vi "_Yt06_Lock.vi"(11 "YTESTER测试数据":T1) -> (3 "YTESTER结论":T2)   [LabVIEW 2017]
doc: "VIClassID=YT_SSTEPFLAG_LOCK\nVIDescription=锁"
uses:
  YtCommon.lvlibp/yt`Step StepBaseInput.ctl
  YtCommon.lvlibp/yt`Step StepResult.ctl
  YtCommon.lvlibp/yt`Step TestData.ctl
  YtCommon.lvlibp/yt`Step System Queue.ctl
  Step`s VIs/YYLLGeneric/variable_W.ctl
  YtCommon.lvlibp/yt`Data-Ytester Type Data.ctl
  0f7d8788-236d-43a4-88cb-40465cf95507.vi
  b398933d-6113-41d7-8023-f37935ba96c7.vi
  <vilib>/Utility/error.llb/Clear Errors.vi
  YtCommon.lvlibp/yt`varSystemlib IO Read Variable.vi
  YtCommon.lvlibp
panel:
  in  "YTESTER开放参数":T4={"YTESTER_BaseInput"={"isTest"=TRUE, "isSkip"=FALSE, "StepName"="锁", "OnPass"=enum."Next", "OnFail"=enum."Terminate", "ReTestNumber"=0.0}, "解锁？"=FALSE, "锁名称"="Lock", "超时s"=-1.0}
  # "#yyll 首先这个必须是重入VI"
  # "YT_SSTEPFLAG_LOCK"
  # "#yyll 注意终止测试对解锁的影响"
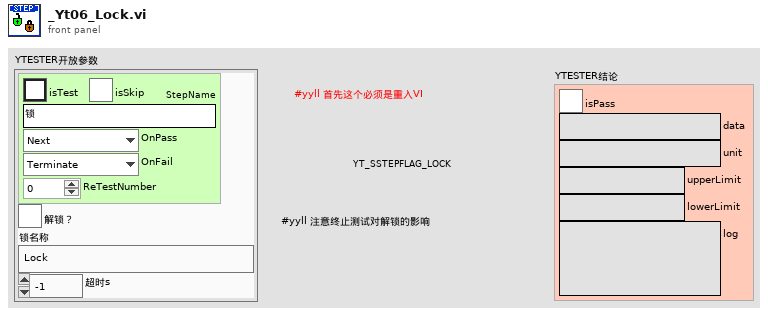
[diagram p1: front panel]
types:
  T1 = typedef "YtCommon.lvlibp/yt`Step TestData.ctl" = cluster{"Socket(From1)":i32, "SN":refnum<notifier>, "StopFlagRef":refnum<notifier>, "YT System Queue":refnum<queue>}
  T2 = typedef "YtCommon.lvlibp/yt`Step StepResult.ctl" = cluster{"isPass":bool, "data":string, "unit":string, "upperLimit":string, "lowerLimit":string, "log":string}
  T3 = typedef "YtCommon.lvlibp/yt`Step StepBaseInput.ctl" = cluster{"isTest":bool, "isSkip":bool, "StepName":string, "OnPass":enum16{"Next", "ToOVER", "Terminate"}, "OnFail":enum16{"Next", "ToOVER", "Terminate"}, "ReTestNumber":dbl}
  T4 = cluster{"YTESTER_BaseInput":T3, "解锁？":bool, "锁名称":string, "超时s":dbl}
  T5 = typedef "variable_W.ctl" = cluster{"YT_TYPE":T6, "TypeData":string[], "Tips":string}
  T6 = typedef "YtCommon.lvlibp/yt`Data-Ytester Type Data.ctl" = enum16{"NULL", "NUM", "BOOL", "TXT", "ENUM", "TIME", "PATH", "VISA", "COMBO", "ColorBox", "RadioBtn", "Array_NUM", "Array_BOOL", "Array_TXT", "Array_ENUM", "Array_PATH", "Array_COMBO"}
  T7 = typedef "YtCommon.lvlibp/yt`Step System Queue.ctl" = cluster{"Socket(From0)":i32, "Cmd":string, "Data":variant}
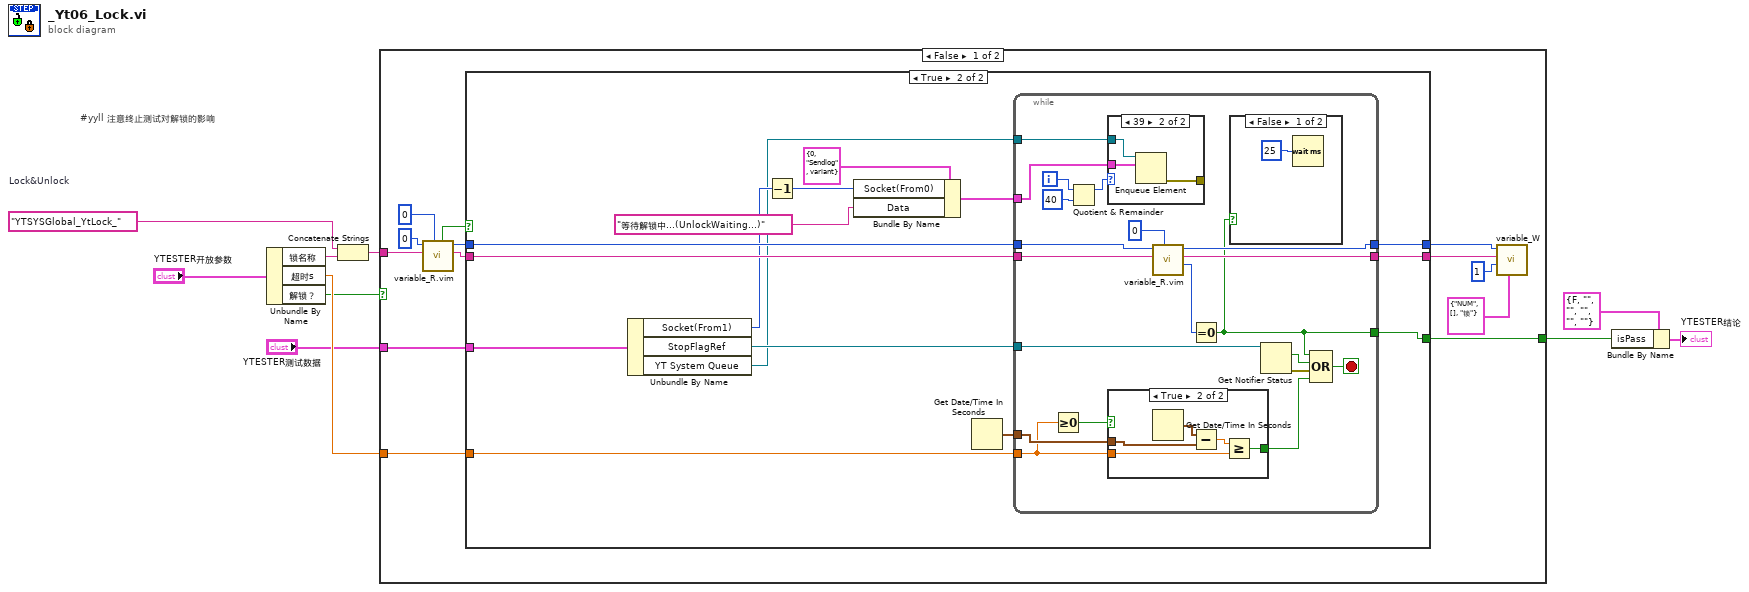
[diagram p0: block diagram]
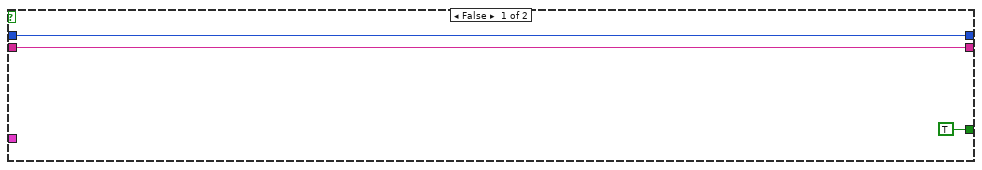
[diagram p2: hidden frame]
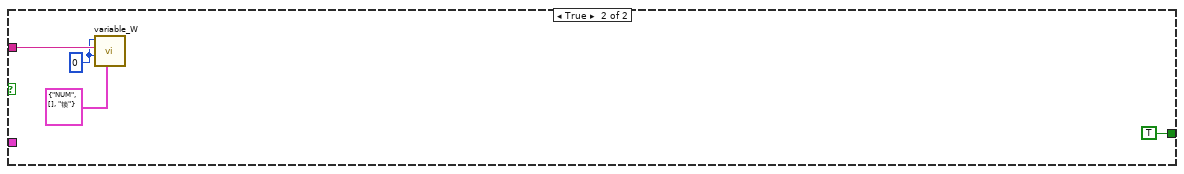
[diagram p6: hidden frame]
diagram:
  w8 = "YTSYSGlobal_YtLock_"  # Lock&Unlock
  # "#yyll 注意终止测试对解锁的影响"
  n1 = Unbundle By Name("YTESTER开放参数") -> ("锁名称"=w1:string, "超时s"=w4:dbl, "解锁？"=w2:bool)
  n2 = Concatenate Strings(w8, w1) -> (w6:string)
  n3 = case shown="False" w2 {
    tunnel: w6 -> [w21 w73]
    tunnel: [w13 TRUE] -> w5
    tunnel: w4 -> [w12 _]
    tunnel: "YTESTER测试数据" -> [w11 _]
    frame False {
      n4 = call "variable_R.vim"("type"=0 ("函数池名称"), "待获取变量名称"=w21, "函数池名称"=0) -> ("待获取变量名out"=w19:string, "函数池名称out"=w20:i32, "found?"=w18:bool)  [unwired: 4 in, 2 out]
      n5 = case shown="True" w18 {
        tunnel: w20 -> [w26 w41]
        tunnel: w19 -> [w25 w40]
        tunnel: [w26 w38] -> w15
        tunnel: [w25 w39] -> w14
        tunnel: [TRUE w37] -> w13
        tunnel: w12 -> [_ w35]
        tunnel: w11 -> [_ w34]
        frame False {
        }
        frame True {
          n6 = Unbundle By Name(w34) -> ("Socket(From1)"=w29:i32, "StopFlagRef"=w33:refnum<notifier>, "YT System Queue"=w27:refnum<queue>)
          n7 = Decrement(x=w29) -> (x-1=w30:i32)
          n8 = Bundle By Name(cluster=T7 {"Socket(From0)"=0, "Cmd"="Sendlog", "Data"=variant} ("element"), "Socket(From0)"=w30, "Data"="等待解锁中...(UnlockWaiting...)" ("Tips")) -> (w28:T7)
          n9 = Get Date/Time In Seconds() -> (seconds since 1Jan1904=w36:timestamp)
          n10 = while {
            tunnel: w41 -> [w61]
            tunnel: w40 -> [w60]
            tunnel: [w57] -> w39
            tunnel: [w56] -> w38
            tunnel: w33 -> [w54]
            tunnel: [w51] -> w37
            tunnel: w36 -> [w49]
            tunnel: w35 -> [w48]
            tunnel: w28 -> [w44]
            tunnel: w27 -> [w43]
            i -> [w42]
            stop <- w52 stop-if-true
            n11 = Greater Or Equal To 0?(x=w48) -> (x >= 0?=w50:bool)
            n12 = Quotient & Remainder(x=w42, y=40) -> (x-y*floor(x/y)=w45:i32)  [unwired: 1 out]
            n13 = case shown="39" w45 {
              tunnel: w43 -> [_ w64]
              tunnel: w44 -> [_ w63]
              tunnel: [_ w62] -> _
              frame 0, Default {
              }
              frame 39 {
                n14 = Enqueue Element(queue=w64, element=w63) -> (error out=w62:errorcluster)  [unwired: 2 in, 2 out]
              }
            }
            n15 = case shown="True" w50 {
              tunnel: w49 -> [_ w68]
              tunnel: w48 -> [_ w66]
              tunnel: [_ w65] -> w47
              frame False {
              }
              frame True {
                n16 = Get Date/Time In Seconds() -> (seconds since 1Jan1904=w69:timestamp)
                n17 = Subtract(x=w69, y=w68) -> (x-y=w67:dbl)
                n18 = Greater Or Equal?(x=w67, y=w66) -> (x >= y?=w65:bool)
              }
            }
            n19 = call "variable_R.vim"("type"=0 ("函数池名称"), "待获取变量名称"=w60, "函数池名称"=w61) -> ("value"=w58:i32, "待获取变量名out"=w57:string, "函数池名称out"=w56:i32)  [unwired: 4 in, 2 out]
            n20 = Equal To 0?(x=w58) -> (x = 0?=w51:bool)
            n21 = case shown="False" w51 {
              frame False {
                n22 = Wait (ms)(milliseconds to wait=u32 25) -> ()  [unwired: 1 out]
              }
              frame True {
              }
            }
            n23 = Get Notifier Status(notifier=w54) -> (current notification=w55:bool, error out=w53:errorcluster)  [unwired: 1 in, 3 out]
            n24 = Compound Arithmetic op=OR(w51, w55, w53, w47) -> (w52:bool)
          }
        }
      }
      n25 = call "variable_W.vi"("附加的Information"=T5 {"YT_TYPE"=enum."NUM", "TypeData"=[], "Tips"="锁"}, "待写入池的输入控件"=1 ("函数池名称"), "待写入池变量名称"=w14, "函数池名称 in"=w15) -> ()  [unwired: 5 in, 3 out]
    }
    frame True {
      w72 = 0 ("函数池名称 in")
      n26 = call "variable_W.vi"("附加的Information"=T5 {"YT_TYPE"=enum."NUM", "TypeData"=[], "Tips"="锁"}, "待写入池的输入控件"=w72, "待写入池变量名称"=w73, "函数池名称 in"=w72) -> ()  [unwired: 5 in, 3 out]
    }
  }
  n27 = Bundle By Name(cluster=T2 {"isPass"=FALSE, "data"="", "unit"="", "upperLimit"="", "lowerLimit"="", "log"=""} ("Result"), "isPass"=w5) -> (→"YTESTER结论":T2)
